vi "DuplicateItem.vi"(8 "error in (no error)":errorcluster, 10 "ItemTag":string, 11 "TreeControl in":refnum<vi>) -> (0 "error out":errorcluster)   [LabVIEW 2020, in "ScriptManager.lvlib"]
uses:
  ScriptManager.lvlib
  lib/UI/TreeControl/TreeControlLib.lvlib
  <vilib>/regexp/Match Regular Expression.xnode
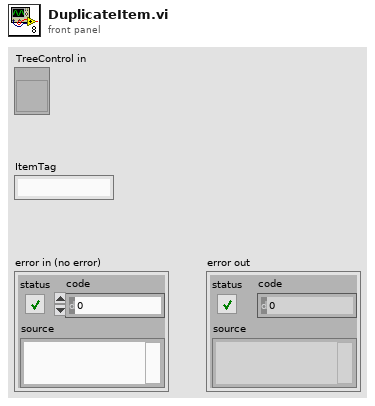
[diagram p1: front panel]
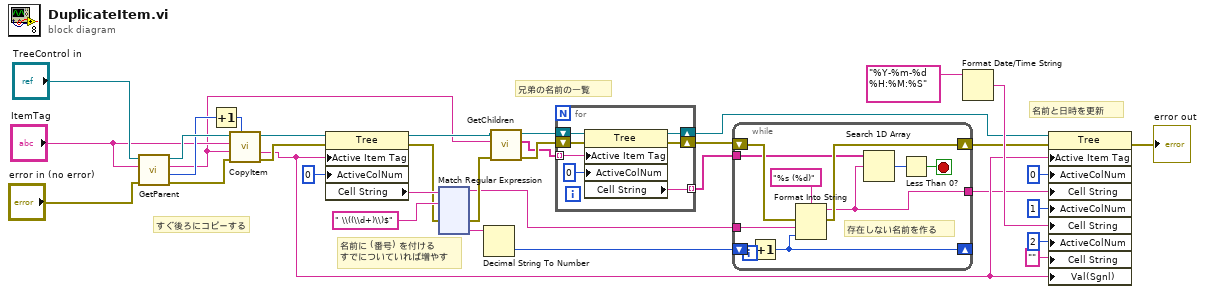
[diagram p0: block diagram]
diagram:
  # "名前と日時を更新"
  # "名前に (番号) を付ける\nすでについていれば増やす"
  # "すぐ後ろにコピーする"
  # "兄弟の名前の一覧"
  n1 = call "GetParent.vi"("error in (no error)"="error in (no error)", "Tag"="ItemTag", "TreeControl in"="TreeControl in") -> ("error out"=w26:errorcluster, "Child Index"=w29:i32, "Parent Tag"=w7:string, "TreeControl out"=w32:refnum<vi>)  [unwired: 5 in]
  n2 = Increment(x=w29) -> (x+1=w30:i32)
  n3 = call "CopyItem.vi"("Insert Inex"=w30, "error in (no error)"=w26, "Parent Tag"=w7, "Source Tag"="ItemTag", "TreeControl in"=w32) -> ("error out"=w34:errorcluster, "Copied Tag"=w13:string, "TreeControl out"=w33:refnum<vi>)  [unwired: 4 in]
  n4 = property class="Tree"(reference=w33, error in=w34, "Active Item Tag"=w13, "ActiveColNum"=0 ("Active Cell:Active Column Number")) -> (reference out=w10:refnum<vi>, error out=w22:errorcluster, "Cell String"=w25:string)
  n5 = xnode "Match Regular Expression"("input string"=w25, "regular expression"=" \\((\\d+)\\)$", "error in"=w22) -> ("before match"=w4:string, "error out"=w9:errorcluster, "submatch 1"=w23:string)  [unwired: 3 in, 3 out]
  n6 = Decimal String To Number(string=w23) -> (number=w21:i32)  [unwired: 2 in, 1 out]
  n7 = call "GetChildren.vi"("error in (no error)"=w9, "Parent Tag"=w7, "TreeControl in"=w10) -> ("error out"=w6:errorcluster, "Children Tag"=w5:string[], "TreeControl out"=w8:refnum<vi>)  [unwired: 6 in]
  n8 = for {
    tunnel: w5 -> [w37] mode=indexing
    shift-right: [w41] -> w2
    shift-left: w8 -> [w42]
    shift-right: [w39] -> w3
    shift-left: w6 -> [w40]
    tunnel: [w36] -> w1 mode=indexing
    n9 = property class="Tree"(reference=w42, error in=w40, "Active Item Tag"=w37, "ActiveColNum"=0 ("Active Cell:Active Column Number")) -> (reference out=w41:refnum<vi>, error out=w39:errorcluster, "Cell String"=w36:string)
  }
  n10 = while {
    shift-right: [w48] -> w17
    shift-left: w3 -> [w52]
    tunnel: w4 -> [w50]
    tunnel: [w43] -> w12
    tunnel: w1 -> [w47]
    shift-right: [w44] -> _
    shift-left: w21 -> [w49]
    stop <- w45 stop-if-true
    # "存在しない名前を作る"
    n11 = Increment(x=w49) -> (x+1=w44:i32)
    n12 = Format Into String(format string="%s (%d)", error in=w52, w50, w44) -> (resulting string=w43:string, error out=w48:errorcluster)  [unwired: 1 in]
    n13 = Search 1D Array(1D array=w47, element=w43) -> (index of element=w46:i32)  [unwired: 1 in]
    n14 = Less Than 0?(x=w46) -> (x < 0?=w45:bool)
  }
  n15 = Format Date/Time String(time format string (%c)="%Y-%m-%d %H:%M:%S") -> (date/time string=w19:string)  [unwired: 2 in]
  n16 = property class="Tree"(reference=w2, error in=w17, "Active Item Tag"=w13, "ActiveColNum"=0 ("Active Cell:Active Column Number"), "Cell String"=w12, "ActiveColNum"=1 ("Active Cell:Active Column Number"), "Cell String"=w19, "ActiveColNum"=2 ("Active Cell:Active Column Number"), "Cell String"="" ("Active Cell:String"), "Val(Sgnl)"=w13) -> (error out=→"error out":errorcluster)  [unwired: 1 out]
